vi "DSF.Execution.Builder.Get Status Pointers.vi"(8 "error in (no error)":errorcluster, 11 "Builder in":refnum<class "DSF.Execution.Builder.lvclass">) -> (0 "error out":errorcluster, 2 "Status Pointers":T1, 3 "Builder out":refnum<class "DSF.Execution.Builder.lvclass">)   [LabVIEW 2016, in "DSF.Engine.lvlib" / "DSF.Execution.Builder.lvclass"]
uses:
  DSF.Execution.Builder.lvclass
  DSF.Execution.Builder.Status Pointers.ctl
  Memory.Pointer/DSF.Memory.Pointer.U32.lvclass
  DSF.Execution.Builder.lvclass/DSF.Execution.Builder.ctl
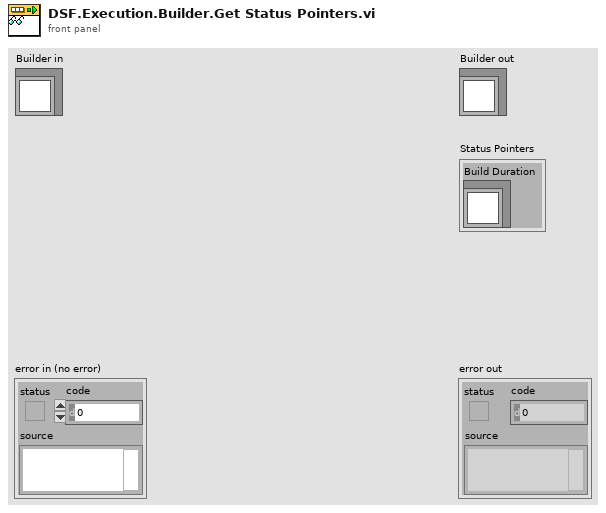
[diagram p1: front panel]
types:
  T1 = typedef "DSF.Engine.lvlib/DSF.Execution.Builder.lvclass/DSF.Execution.Builder.Status Pointers.ctl" = cluster{"Build Duration":refnum<class "DSF.Memory.Pointer.U32.lvclass">}
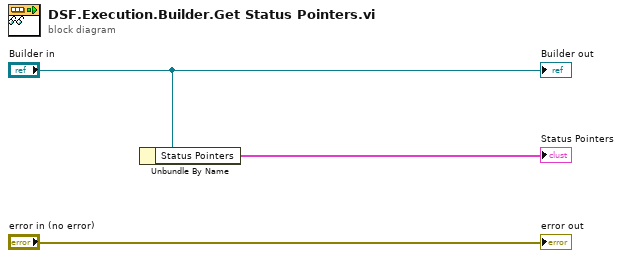
[diagram p0: block diagram]
diagram:
  n1 = Unbundle By Name("Builder in") -> ("Status Pointers"=→"Status Pointers":T1)
  "error out" <- "error in (no error)"
  "Builder out" <- "Builder in"
